vi "PVCAM_OpenCamera.vi"(8 "error in (no error)":errorcluster, 9 "mode":i16, 11 "cameraName":string) -> (0 "error out":errorcluster, 1 "return out":i16, 3 "hCam out":i16)   [LabVIEW 2021]
uses:
  pvcam64.dll
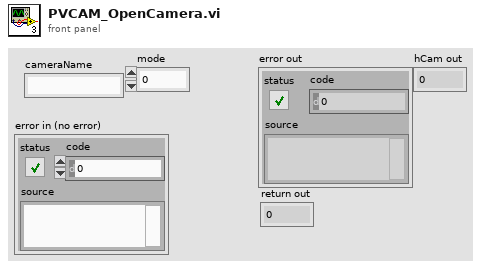
[diagram p1: front panel]
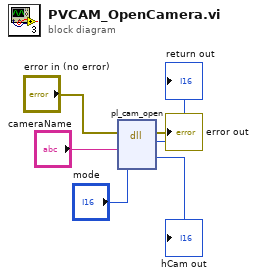
[diagram p0: block diagram]
diagram:
  n1 = dll-call lib="pvcam64.dll" fn="pl_cam_open"(error in="error in (no error)", "cameraName"="cameraName", "mode"="mode") -> (error out=→"error out":errorcluster, "return type"=→"return out":i16, "hCam"=→"hCam out":i16)  [unwired: 5 in, 1 out]
